vi "Autonomous Independent.vi"() -> ()   [LabVIEW 2011]
doc: "This VI is called when autonomous begins, and will automatically be terminated when autonomous ends. You can carry out timed or sensor driven robot movement independently without needing to return to the caller."
uses:
  <vilib>/Rock Robotics/WPI/Relay/WPI_RelayValue.ctl
  Robot Global Data.vi
  PID Set Points.vi
panel:
  out "Numeric 2":i32
  out "Numeric":dbl
  in  "Autonomous Type":T1(radio)
  # "Auto 1: Timed. Drive Forward. From Center\nAuto 2: Shoot from Key w Indexer\nAuto 3: Camera: Stationary. From Center\nAuto 4: Camera: Stationary. From Right\nAuto 5: Camera: Drive Up. Ceter\nAuto 6: Camera: Drive Up. Right"
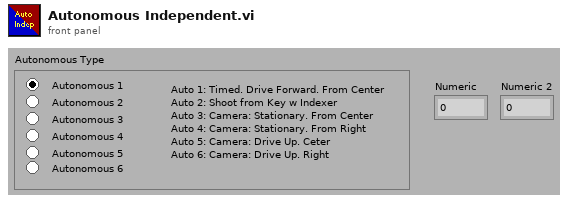
[diagram p1: front panel]
types:
  T1 = enum32{"Autonomous 1", "Autonomous 2", "Autonomous 4", "Autonomous 3", "Autonomous 5", "Autonomous 6"}
  T2 = typedef "WPI_RobotDriveDevRef.ctl" = cluster{"DevStatus":errorcluster, "Motors[]":T3[], "Square Inputs":bool, "Max Output":dbl, "Isochronous":bool}
  T3 = typedef "WPI_MotorControlDeviceRef.ctl" = cluster{"DeviceStatus":errorcluster, "Type":enum16{"PWM", "CAN"}, "PWM":cluster{"Digital Module":T4, "PWM Channel":T5, "DeadBand":T6}, "CAN":cluster{"Device Number":u8, "Control Mode":T7, "Semaphore":T8, "Max Vout":dbl}, "Invert":bool, "TransformRef":T9, "InvTransformRef":T9}
  T4 = typedef "FPGA_TypedefDigitalModule.ctl" = enum16{"Digital Module 1", "Digital Module 2"}
  T5 = typedef "FPGA_DIOPWMChannel.ctl" = enum8{"PWM 1", "PWM 2", "PWM 3", "PWM 4", "PWM 5", "PWM 6", "PWM 7", "PWM 8", "PWM 9", "PWM 10", "Invalid"}
  T6 = typedef "WPI_PWMDeadband.ctl" = cluster{"Name":string, "maxPositivePwm":i32, "minPositivePwm":i32, "centerPwm":i32, "maxNegativePwm":i32, "minNegativePwm":i32, "angularRange":u16}
  T7 = typedef "WPI_CANJaguar_ControlMode.ctl" = enum8{"Percent VBus", "Current", "Speed", "Position", "Voltage"}
  T8 = typedef "Semaphore RefNum" = refnum<k1>
  T9 = typedef "WPI_PWMTransform_ConPane.ctl" = refnum<vi>
  T10 = typedef "WPI_EncoderDevRef.ctl" = cluster{"DevStatus":errorcluster, "EncoderIndex":T11, "CounterIndex":T12, "DistancePerCount":dbl, "Decoding Type":T13}
  T11 = typedef "FPGA_EncoderIdx.ctl" = enum8{"Enc 0", "Enc 1", "Enc 2", "Enc 3", "Invalid"}
  T12 = typedef "FPGA_CounterCtrSystemIndex.ctl" = enum8{"Ctr 0", "Ctr 1", "Ctr 2", "Ctr 3", "Ctr 4", "Ctr 5", "Ctr 6", "Ctr 7", "Invalid"}
  T13 = typedef "WPI_EncoderType.ctl" = enum16{"1x", "2x", "4x"}
  T14 = typedef "WPI_RelayValue.ctl" = enum16{"Off", "On", "Forward", "Reverse"}
  T15 = cluster{"Position":cluster{"X":dbl, "Y":dbl}, "Distance (ft)":dbl}[]
  T16 = cluster{"Position":cluster{"X":dbl, "Y":dbl}, "Distance (ft)":dbl}
  T17 = typedef "WPI_RelayDevRef.ctl" = cluster{"DevStatus":errorcluster, "Relay Channel":T18, "Digital Module":T4, "Relay Direction":T19}
  T18 = typedef "FPGA_DIORelayChannel.ctl" = enum8{"Relay 1", "Relay 2", "Relay 3", "Relay 4", "Relay 5", "Relay 6", "Relay 7", "Relay 8", "Invalid"}
  T19 = typedef "WPI_RelayDirection.ctl" = enum16{"Both directions", "Forward only", "Reverse only"}
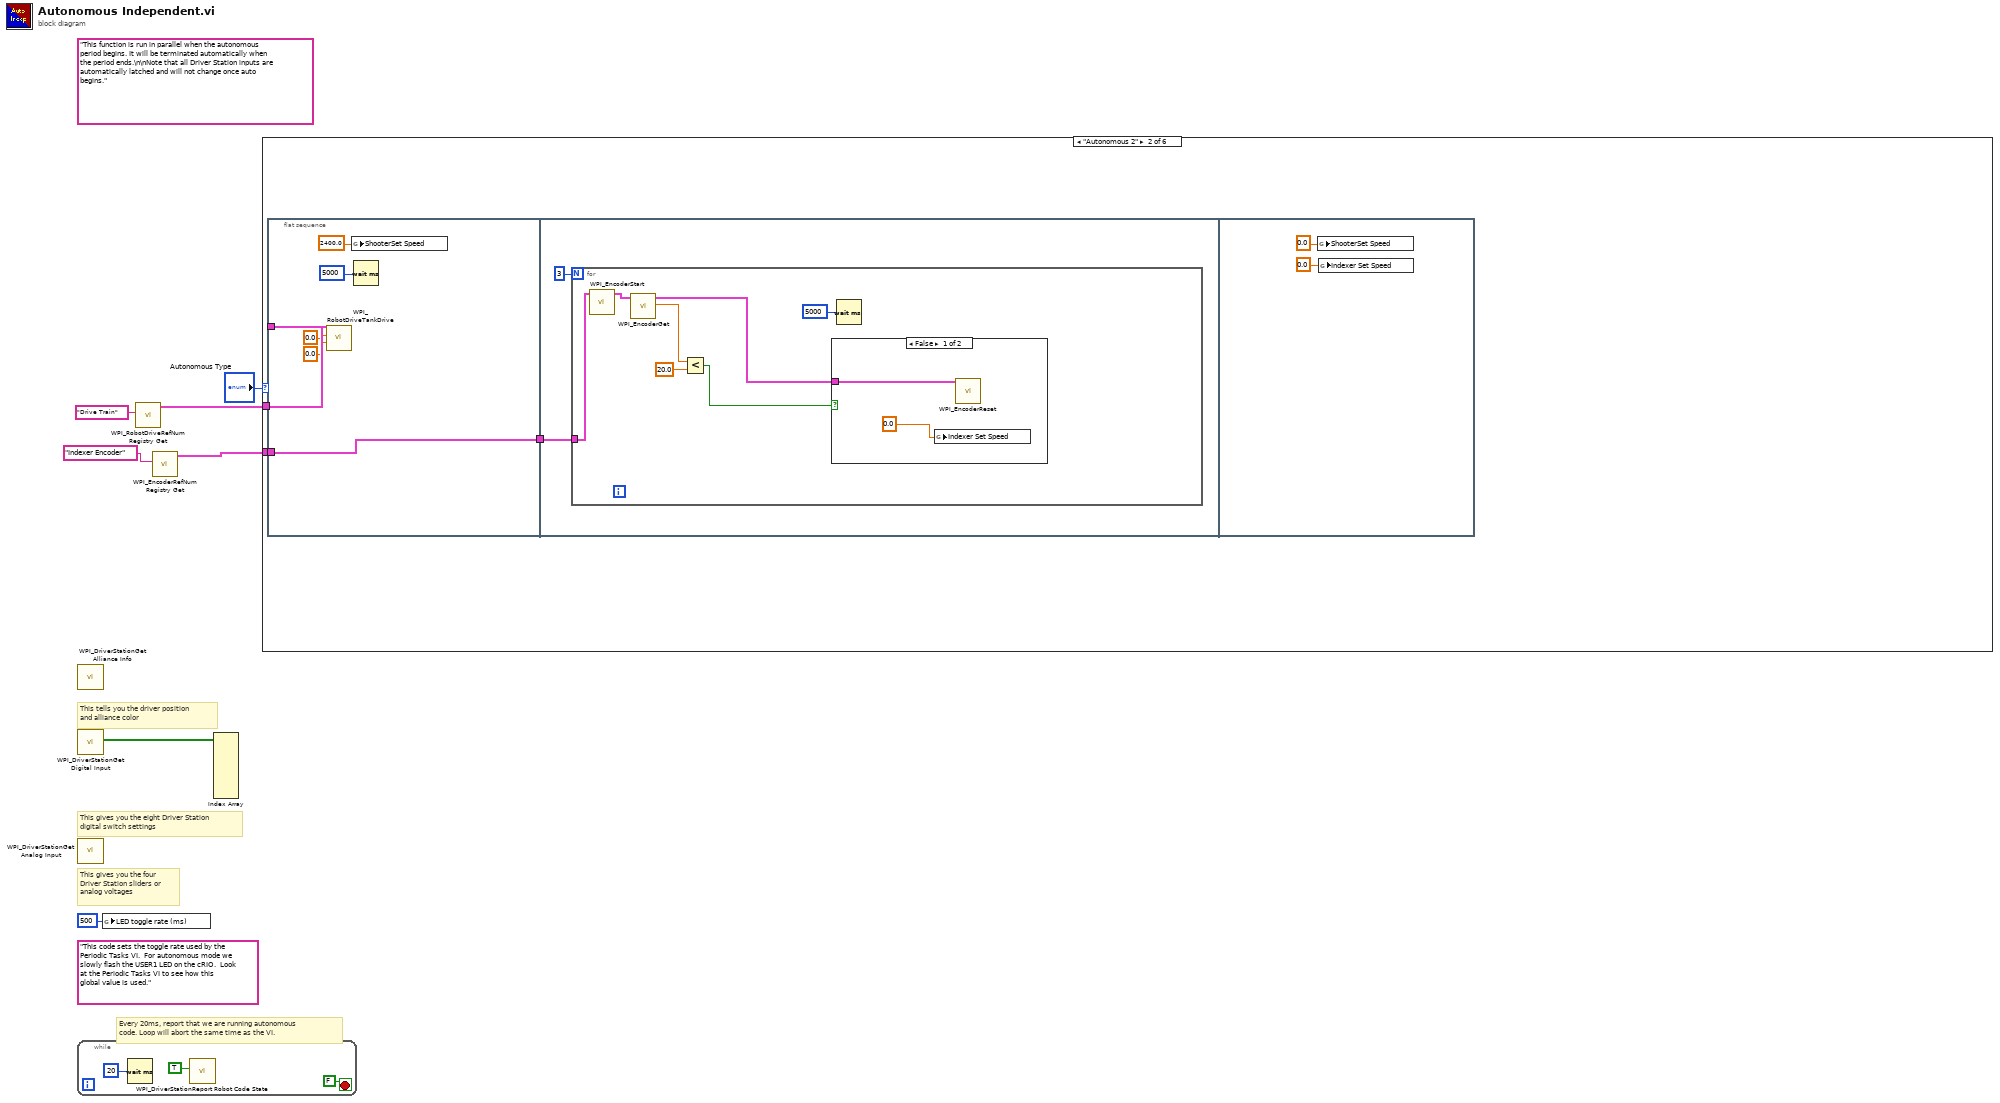
[diagram p0: block diagram]
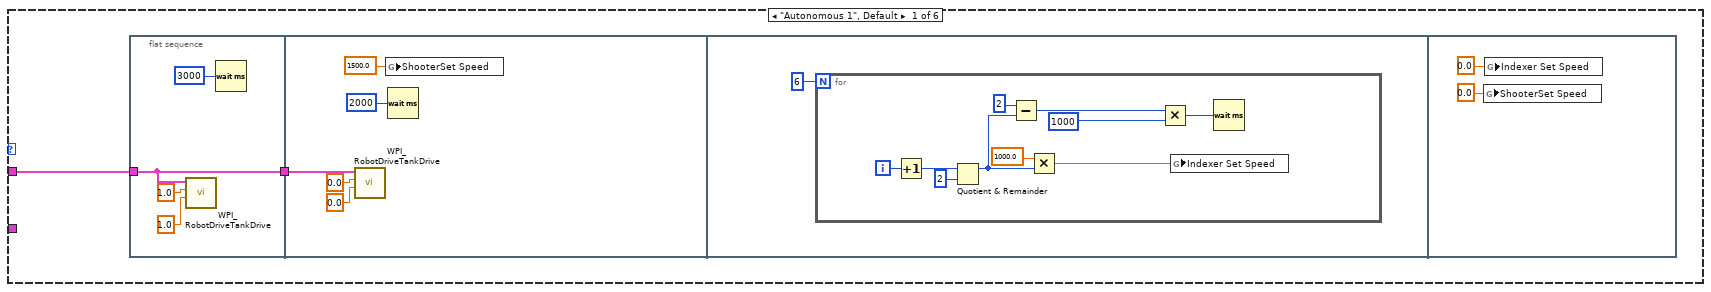
[diagram p2: hidden frame]
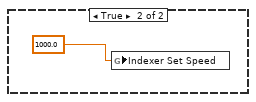
[diagram p3: hidden frame]
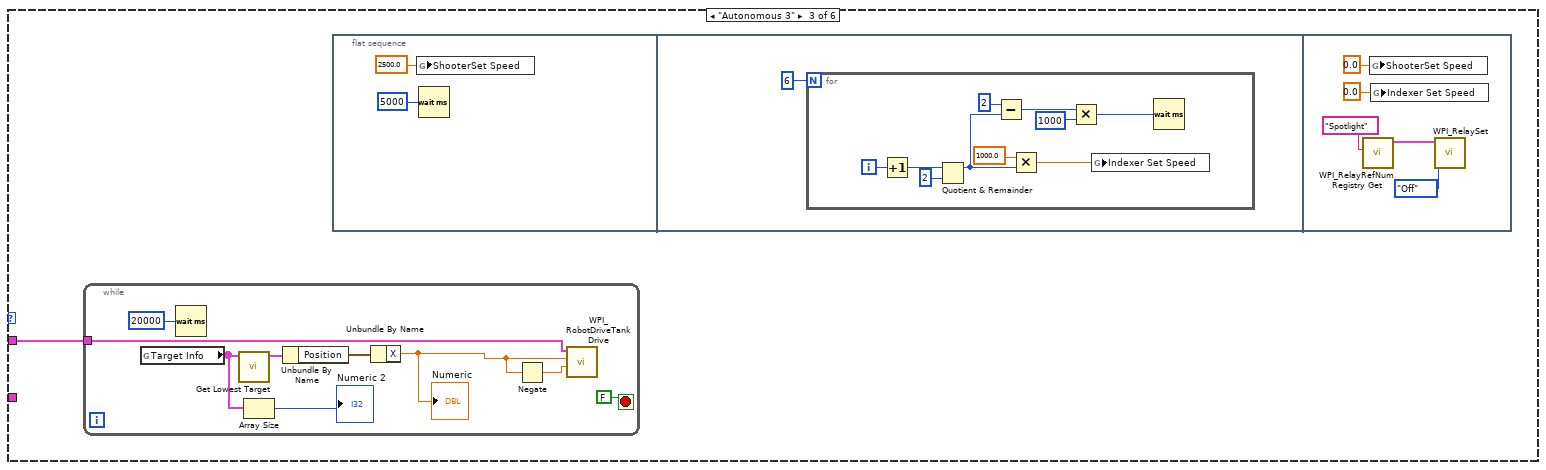
[diagram p4: hidden frame]
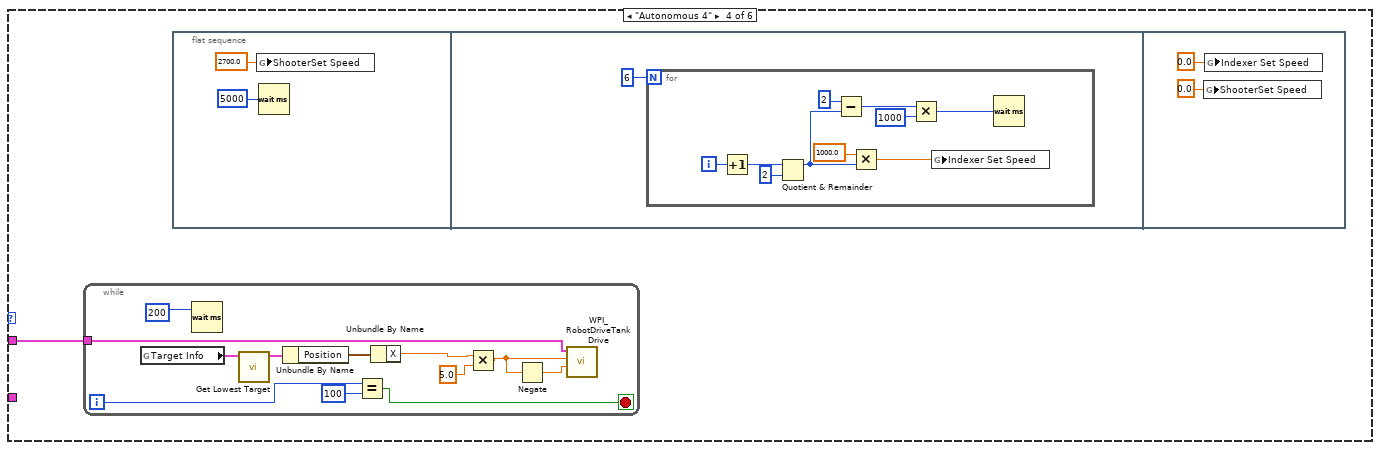
[diagram p5: hidden frame]
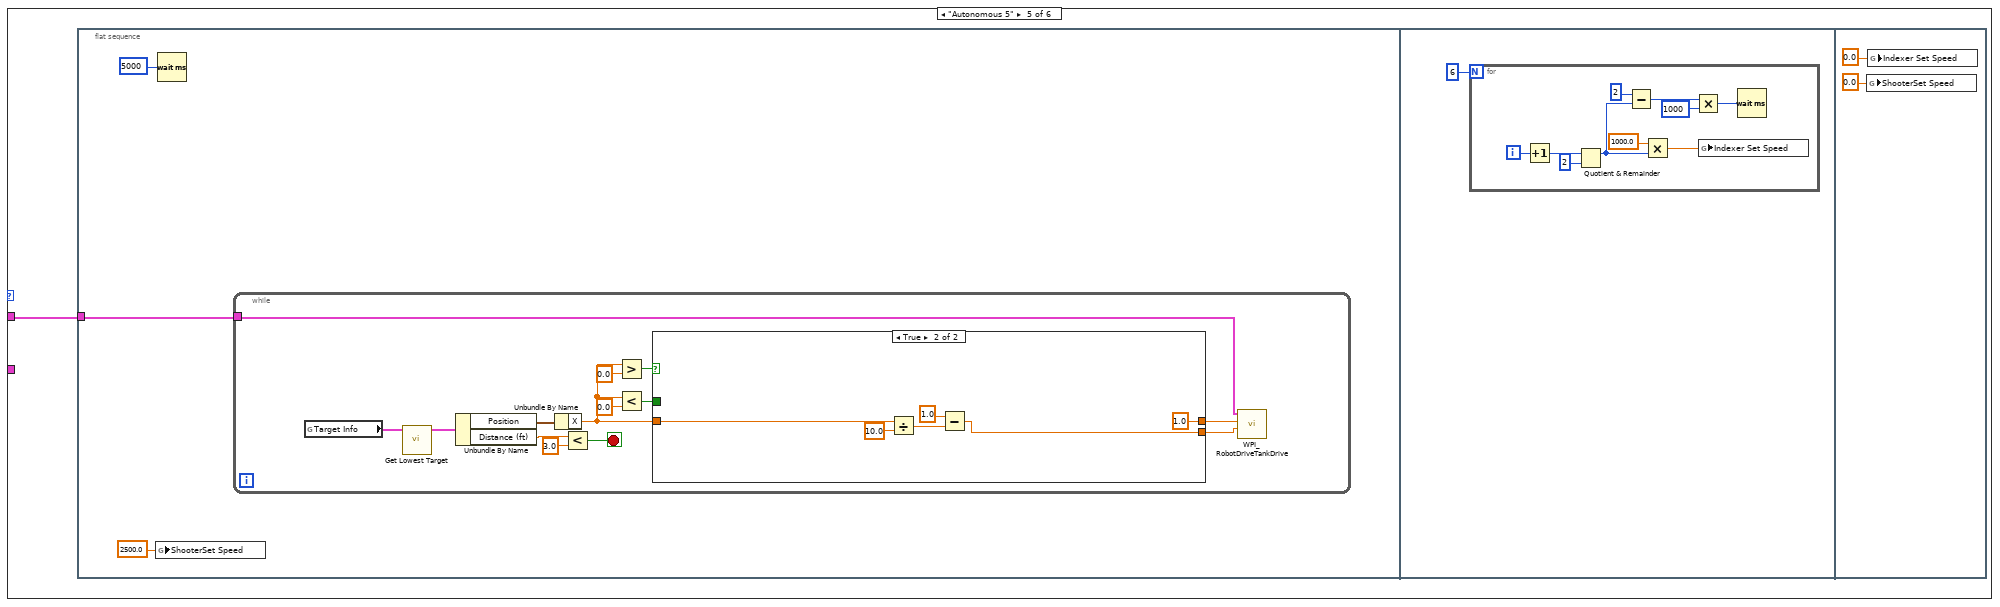
[diagram p6: hidden frame]
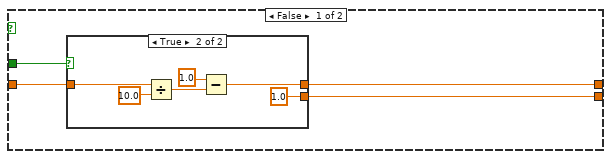
[diagram p7: hidden frame]
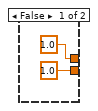
[diagram p8: hidden frame]
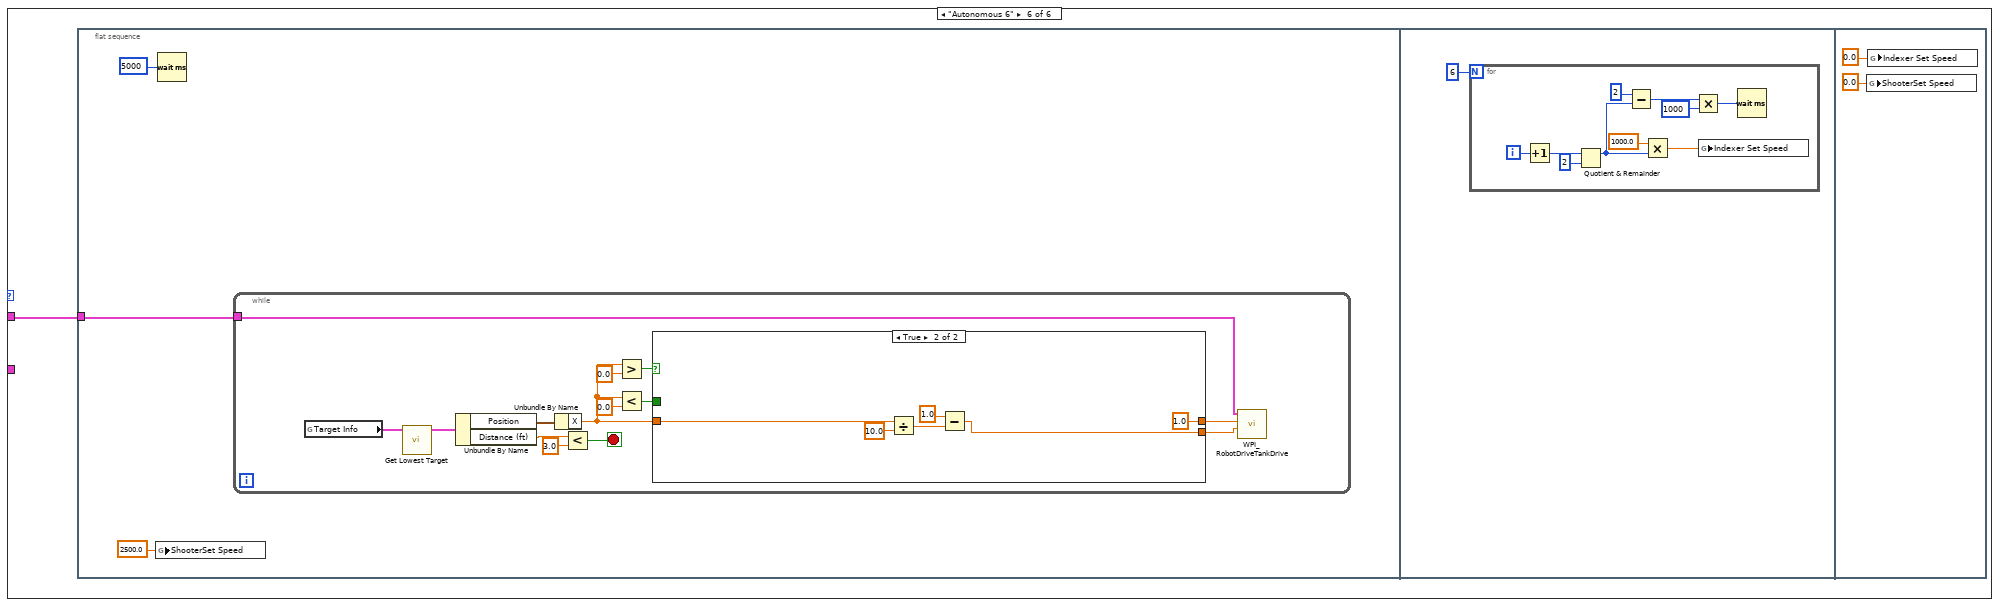
[diagram p9: hidden frame]
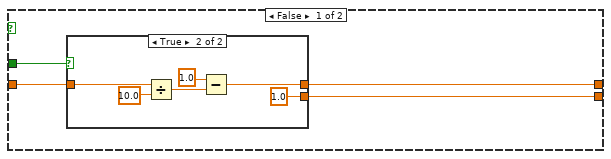
[diagram p10: hidden frame]
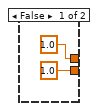
[diagram p11: hidden frame]
diagram:
  (unwired) "This code sets the toggle rate used by the Periodic Tasks VI.  For autonomous mode we slowly flash the USER1 LED on the cRIO.  Look at the Periodic Tasks VI to see how this global value is used."
  (unwired) "This function is run in parallel when the autonomous period begins. It will be terminated automatically when the period ends.\n\nNote that all Driver Station inputs are automatically latched and will not change once auto begins."
  # "Every 20ms, report that we are running autonomous\ncode. Loop will abort the same time as the VI."
  # "This tells you the driver position\nand alliance color"
  # "This gives you the eight Driver Station\ndigital switch settings"
  # "This gives you the four\nDriver Station sliders or\nanalog voltages"
  n1 = call <vilib>:"WPI_DriverStationGet Alliance Info.vi"() -> ()  [unwired: 12 out]
  n2 = call <vilib>:"WPI_DriverStationGet Digital Input.vi"() -> ("Driver Station Digital Input (1-8)"=w7:bool[])  [unwired: 11 out]
  n3 = call <vilib>:"WPI_DriverStationGet Analog Input.vi"() -> ()  [unwired: 12 out]
  n4 = while {
    stop <- FALSE stop-if-true
    n5 = Wait (ms)(milliseconds to wait=u32 20) -> ()  [unwired: 1 out]
    n6 = call <vilib>:"WPI_DriverStationReport Robot Code State.vi"("Autonomous"=TRUE) -> ()  [unwired: 10 in, 1 out]
  }
  n7 = global write "Robot Global Data.vi" "LED toggle rate (ms)"(u32 500 ("LED ms toggle rate")) -> ()
  n8 = call <vilib>:"WPI_RobotDriveRefNum Registry Get.vi"("refnum name"="Drive Train") -> ("RobotDriveDevRef"=w3:T2)  [unwired: 9 in, 1 out]
  n9 = call <vilib>:"WPI_EncoderRefNum Registry Get.vi"("refnum name"="Indexer Encoder") -> ("EncoderDevRef"=w1:T10)  [unwired: 9 in, 1 out]
  n10 = Index Array(array=w7) -> ()  [unwired: 8 in, 8 out]
  n11 = case shown="\"Autonomous 2\"" "Autonomous Type" {
    tunnel: w3 -> [w12 w37 w58 w86 w114 w163]
    tunnel: w1 -> [_ w36 _ _ _ _]
    frame "Autonomous 1", Default {
      n12 = flat-sequence {
        tunnel: w12 -> [w16]
        tunnel: [w16] -> w11
        tunnel: w11 -> [w21]
        frame #0 {
          n13 = call <vilib>:"WPI_RobotDriveTankDrive.vi"("Right axis value"=1.0, "Left axis value"=1.0, "RobotDriveDevRef"=w16) -> ()  [unwired: 7 in, 2 out]
          n14 = Wait (ms)(milliseconds to wait=u32 3000) -> ()  [unwired: 1 out]
        }
        frame #1 {
          n15 = call <vilib>:"WPI_RobotDriveTankDrive.vi"("Right axis value"=0.0, "Left axis value"=0.0, "RobotDriveDevRef"=w21) -> ()  [unwired: 7 in, 2 out]
          n16 = global write "PID Set Points.vi" "ShooterSet Speed"(1500.0 ("ShooterSet Speed")) -> ()
          n17 = Wait (ms)(milliseconds to wait=u32 2000) -> ()  [unwired: 1 out]
        }
        frame #2 {
          n18 = for {
            N: 6 -> [_]
            i -> [w29]
            n19 = Increment(x=w29) -> (x+1=w28:i32)
            n20 = Quotient & Remainder(x=w28, y=2) -> (x-y*floor(x/y)=w26:i32)  [unwired: 1 out]
            n21 = Subtract(x=2, y=w26) -> (x-y=w25:i32)
            n22 = Multiply(x=1000.0, y=w26) -> (x*y=w30:dbl)
            n23 = Multiply(x=w25, y=1000 ("x")) -> (x*y=w23:i32)
            n24 = global write "PID Set Points.vi" "Indexer Set Speed"(w30) -> ()
            n25 = Wait (ms)(milliseconds to wait=w23) -> ()  [unwired: 1 out]
          }
        }
        frame #3 {
          n26 = global write "PID Set Points.vi" "ShooterSet Speed"(0.0 ("ShooterSet Speed")) -> ()
          n27 = global write "PID Set Points.vi" "Indexer Set Speed"(0.0 ("Indexer Set Speed")) -> ()
        }
      }
    }
    frame "Autonomous 2" {
      n28 = flat-sequence {
        tunnel: w37 -> [w39]
        tunnel: w36 -> [w38]
        tunnel: [w38] -> w35
        tunnel: w35 -> [w44]
        frame #0 {
          n29 = call <vilib>:"WPI_RobotDriveTankDrive.vi"("Right axis value"=0.0, "Left axis value"=0.0, "RobotDriveDevRef"=w39) -> ()  [unwired: 7 in, 2 out]
          n30 = global write "PID Set Points.vi" "ShooterSet Speed"(2400.0 ("ShooterSet Speed")) -> ()
          n31 = Wait (ms)(milliseconds to wait=u32 5000) -> ()  [unwired: 1 out]
        }
        frame #1 {
          n32 = for {
            N: 3 -> [_]
            tunnel: w44 -> [w47]
            n33 = call <vilib>:"WPI_EncoderStart.vi"("EncoderDevRef"=w47) -> ("EncoderDevRef"=w48:T10)  [unwired: 9 in, 1 out]
            n34 = call <vilib>:"WPI_EncoderGet.vi"("EncoderDevRef"=w48) -> ("Distance"=w49:dbl, "EncoderDevRef"=w46:T10)  [unwired: 5 in, 4 out]
            n35 = Less?(x=w49, y=20.0) -> (x < y?=w51:bool)
            n36 = case shown="False" w51 {
              tunnel: w46 -> [w53 _]
              frame False {
                n37 = global write "PID Set Points.vi" "Indexer Set Speed"(0.0 ("Indexer Set Speed")) -> ()
                n38 = call <vilib>:"WPI_EncoderReset.vi"("EncoderDevRef"=w53) -> ()  [unwired: 9 in, 2 out]
              }
              frame True {
                n39 = global write "PID Set Points.vi" "Indexer Set Speed"(1000.0 ("Indexer Set Speed")) -> ()
              }
            }
            n40 = Wait (ms)(milliseconds to wait=u32 5000) -> ()  [unwired: 1 out]
          }
        }
        frame #2 {
          n41 = global write "PID Set Points.vi" "ShooterSet Speed"(0.0 ("ShooterSet Speed")) -> ()
          n42 = global write "PID Set Points.vi" "Indexer Set Speed"(0.0 ("Indexer Set Speed")) -> ()
        }
      }
    }
    frame "Autonomous 3" {
      n43 = while {
        tunnel: w58 -> [w84]
        stop <- FALSE stop-if-true
        n44 = global read "Robot Global Data.vi" "Target Info"() -> (w78:T15)
        n45 = Wait (ms)(milliseconds to wait=u32 20000) -> ()  [unwired: 1 out]
        n46 = call "Get Lowest Target.vi"("Target Info"=w78) -> ("Cluster"=w81:T16)  [unwired: 10 in]
        n47 = Array Size(array=w78) -> (size(s)=→"Numeric 2":i32)
        n48 = Unbundle By Name(w81) -> ("Position"=w83:cluster{"X":dbl, "Y":dbl})
        n49 = Unbundle By Name(w83) -> ("X"=w79:dbl)
        "Numeric" <- w79
        n50 = Negate(x=w79) -> (-x=w82:dbl)
        n51 = call <vilib>:"WPI_RobotDriveTankDrive.vi"("Right axis value"=w82, "Left axis value"=w79, "RobotDriveDevRef"=w84) -> ()  [unwired: 7 in, 2 out]
      }
      n52 = flat-sequence {
        frame #0 {
          n53 = global write "PID Set Points.vi" "ShooterSet Speed"(2500.0 ("ShooterSet Speed")) -> ()
          n54 = Wait (ms)(milliseconds to wait=u32 5000) -> ()  [unwired: 1 out]
        }
        frame #1 {
          n55 = for {
            N: 6 -> [_]
            i -> [w68]
            n56 = Increment(x=w68) -> (x+1=w67:i32)
            n57 = Quotient & Remainder(x=w67, y=2) -> (x-y*floor(x/y)=w65:i32)  [unwired: 1 out]
            n58 = Subtract(x=2, y=w65) -> (x-y=w64:i32)
            n59 = Multiply(x=1000.0, y=w65) -> (x*y=w69:dbl)
            n60 = Multiply(x=w64, y=1000 ("x")) -> (x*y=w62:i32)
            n61 = global write "PID Set Points.vi" "Indexer Set Speed"(w69) -> ()
            n62 = Wait (ms)(milliseconds to wait=w62) -> ()  [unwired: 1 out]
          }
        }
        frame #2 {
          n63 = call <vilib>:"WPI_RelayRefNum Registry Get.vi"("refnum name"="Spotlight") -> ("RelayDevRef"=w73:T17)  [unwired: 9 in, 1 out]
          n64 = global write "PID Set Points.vi" "ShooterSet Speed"(0.0 ("ShooterSet Speed")) -> ()
          n65 = global write "PID Set Points.vi" "Indexer Set Speed"(0.0 ("ShooterSet Speed")) -> ()
          n66 = call <vilib>:"WPI_RelaySet.vi"("RelayValue"=WPI_RelayValue."Off", "RelayDevRef"=w73) -> ()  [unwired: 8 in, 2 out]
        }
      }
    }
    frame "Autonomous 4" {
      n67 = while {
        tunnel: w86 -> [w112]
        i -> [w104]
        stop <- w102 stop-if-true
        n68 = global read "Robot Global Data.vi" "Target Info"() -> (w109:T15)
        n69 = Wait (ms)(milliseconds to wait=u32 200) -> ()  [unwired: 1 out]
        n70 = call "Get Lowest Target.vi"("Target Info"=w109) -> ("Cluster"=w108:T16)  [unwired: 10 in]
        n71 = Unbundle By Name(w108) -> ("Position"=w111:cluster{"X":dbl, "Y":dbl})
        n72 = Equal?(x=w104, y=100) -> (x = y?=w102:bool)
        n73 = Unbundle By Name(w111) -> ("X"=w107:dbl)
        n74 = Multiply(x=w107, y=5.0) -> (x*y=w105:dbl)
        n75 = Negate(x=w105) -> (-x=w110:dbl)
        n76 = call <vilib>:"WPI_RobotDriveTankDrive.vi"("Right axis value"=w110, "Left axis value"=w105, "RobotDriveDevRef"=w112) -> ()  [unwired: 7 in, 2 out]
      }
      n77 = flat-sequence {
        frame #0 {
          n78 = global write "PID Set Points.vi" "ShooterSet Speed"(2700.0 ("ShooterSet Speed")) -> ()
          n79 = Wait (ms)(milliseconds to wait=u32 5000) -> ()  [unwired: 1 out]
        }
        frame #1 {
          n80 = for {
            N: 6 -> [_]
            i -> [w96]
            n81 = Increment(x=w96) -> (x+1=w95:i32)
            n82 = Quotient & Remainder(x=w95, y=2) -> (x-y*floor(x/y)=w93:i32)  [unwired: 1 out]
            n83 = Subtract(x=2, y=w93) -> (x-y=w92:i32)
            n84 = Multiply(x=1000.0, y=w93) -> (x*y=w97:dbl)
            n85 = Multiply(x=w92, y=1000 ("x")) -> (x*y=w90:i32)
            n86 = global write "PID Set Points.vi" "Indexer Set Speed"(w97) -> ()
            n87 = Wait (ms)(milliseconds to wait=w90) -> ()  [unwired: 1 out]
          }
        }
        frame #2 {
          n88 = global write "PID Set Points.vi" "ShooterSet Speed"(0.0 ("ShooterSet Speed")) -> ()
          n89 = global write "PID Set Points.vi" "Indexer Set Speed"(0.0 ("ShooterSet Speed")) -> ()
        }
      }
    }
    frame "Autonomous 5" {
      n90 = flat-sequence {
        tunnel: w114 -> [w117]
        frame #0 {
          n91 = global write "PID Set Points.vi" "ShooterSet Speed"(2500.0 ("ShooterSet Speed")) -> ()
          n92 = Wait (ms)(milliseconds to wait=u32 5000) -> ()  [unwired: 1 out]
          n93 = while {
            tunnel: w117 -> [w128]
            stop <- w118 stop-if-true
            n94 = global read "Robot Global Data.vi" "Target Info"() -> (w131:T15)
            n95 = call "Get Lowest Target.vi"("Target Info"=w131) -> ("Cluster"=w130:T16)  [unwired: 10 in]
            n96 = Unbundle By Name(w130) -> ("Position"=w129:cluster{"X":dbl, "Y":dbl}, "Distance (ft)"=w120:dbl)
            n97 = Unbundle By Name(w129) -> ("X"=w123:dbl)
            n98 = Less?(x=w120, y=3.0) -> (x < y?=w118:bool)
            n99 = Greater?(x=w123, y=0.0) -> (0:w126:bool)
            n100 = Less?(x=w123, y=0.0) -> (x < y?=w121:bool)
            n101 = case shown="True" w126 {
              tunnel: w123 -> [w134 w148]
              tunnel: [w132 w145] -> w124
              tunnel: [w133 1.0] -> w125
              tunnel: w121 -> [w135 _]
              frame False {
                n102 = case shown="True" w135 {
                  tunnel: w134 -> [_ w140]
                  tunnel: [1.0 w139] -> w133
                  tunnel: [1.0 1.0] -> w132
                  frame False {
                  }
                  frame True {
                    n103 = Divide(x=w140, y=10.0) -> (x/y=w141:dbl)
                    n104 = Subtract(x=1.0, y=w141) -> (x-y=w139:dbl)
                  }
                }
              }
              frame True {
                n105 = Divide(x=w148, y=10.0) -> (x/y=w146:dbl)
                n106 = Subtract(x=1.0, y=w146) -> (x-y=w145:dbl)
              }
            }
            n107 = call <vilib>:"WPI_RobotDriveTankDrive.vi"("Right axis value"=w124, "Left axis value"=w125, "RobotDriveDevRef"=w128) -> ()  [unwired: 7 in, 2 out]
          }
        }
        frame #1 {
          n108 = for {
            N: 6 -> [_]
            i -> [w157]
            n109 = Increment(x=w157) -> (x+1=w156:i32)
            n110 = Quotient & Remainder(x=w156, y=2) -> (x-y*floor(x/y)=w154:i32)  [unwired: 1 out]
            n111 = Subtract(x=2, y=w154) -> (x-y=w153:i32)
            n112 = Multiply(x=1000.0, y=w154) -> (x*y=w158:dbl)
            n113 = Multiply(x=w153, y=1000 ("x")) -> (x*y=w151:i32)
            n114 = global write "PID Set Points.vi" "Indexer Set Speed"(w158) -> ()
            n115 = Wait (ms)(milliseconds to wait=w151) -> ()  [unwired: 1 out]
          }
        }
        frame #2 {
          n116 = global write "PID Set Points.vi" "ShooterSet Speed"(0.0 ("ShooterSet Speed")) -> ()
          n117 = global write "PID Set Points.vi" "Indexer Set Speed"(0.0 ("ShooterSet Speed")) -> ()
        }
      }
    }
    frame "Autonomous 6" {
      n118 = flat-sequence {
        tunnel: w163 -> [w166]
        frame #0 {
          n119 = global write "PID Set Points.vi" "ShooterSet Speed"(2500.0 ("ShooterSet Speed")) -> ()
          n120 = Wait (ms)(milliseconds to wait=u32 5000) -> ()  [unwired: 1 out]
          n121 = while {
            tunnel: w166 -> [w177]
            stop <- w167 stop-if-true
            n122 = global read "Robot Global Data.vi" "Target Info"() -> (w180:T15)
            n123 = call "Get Lowest Target.vi"("Target Info"=w180) -> ("Cluster"=w179:T16)  [unwired: 10 in]
            n124 = Unbundle By Name(w179) -> ("Position"=w178:cluster{"X":dbl, "Y":dbl}, "Distance (ft)"=w169:dbl)
            n125 = Unbundle By Name(w178) -> ("X"=w172:dbl)
            n126 = Less?(x=w169, y=3.0) -> (x < y?=w167:bool)
            n127 = Greater?(x=w172, y=0.0) -> (0:w175:bool)
            n128 = Less?(x=w172, y=0.0) -> (x < y?=w170:bool)
            n129 = case shown="True" w175 {
              tunnel: w172 -> [w183 w197]
              tunnel: [w181 w194] -> w173
              tunnel: [w182 1.0] -> w174
              tunnel: w170 -> [w184 _]
              frame False {
                n130 = case shown="True" w184 {
                  tunnel: w183 -> [_ w189]
                  tunnel: [1.0 w188] -> w182
                  tunnel: [1.0 1.0] -> w181
                  frame False {
                  }
                  frame True {
                    n131 = Divide(x=w189, y=10.0) -> (x/y=w190:dbl)
                    n132 = Subtract(x=1.0, y=w190) -> (x-y=w188:dbl)
                  }
                }
              }
              frame True {
                n133 = Divide(x=w197, y=10.0) -> (x/y=w195:dbl)
                n134 = Subtract(x=1.0, y=w195) -> (x-y=w194:dbl)
              }
            }
            n135 = call <vilib>:"WPI_RobotDriveTankDrive.vi"("Right axis value"=w173, "Left axis value"=w174, "RobotDriveDevRef"=w177) -> ()  [unwired: 7 in, 2 out]
          }
        }
        frame #1 {
          n136 = for {
            N: 6 -> [_]
            i -> [w206]
            n137 = Increment(x=w206) -> (x+1=w205:i32)
            n138 = Quotient & Remainder(x=w205, y=2) -> (x-y*floor(x/y)=w203:i32)  [unwired: 1 out]
            n139 = Subtract(x=2, y=w203) -> (x-y=w202:i32)
            n140 = Multiply(x=1000.0, y=w203) -> (x*y=w207:dbl)
            n141 = Multiply(x=w202, y=1000 ("x")) -> (x*y=w200:i32)
            n142 = global write "PID Set Points.vi" "Indexer Set Speed"(w207) -> ()
            n143 = Wait (ms)(milliseconds to wait=w200) -> ()  [unwired: 1 out]
          }
        }
        frame #2 {
          n144 = global write "PID Set Points.vi" "ShooterSet Speed"(0.0 ("ShooterSet Speed")) -> ()
          n145 = global write "PID Set Points.vi" "Indexer Set Speed"(0.0 ("ShooterSet Speed")) -> ()
        }
      }
    }
  }
